vi "TxtToEye.vi"() -> ()   [LabVIEW 2022 SP3]
uses:
  <vilib>/Utility/file.llb/Read From Spreadsheet File (DBL).vi
  <vilib>/Analysis/NI_AALBase.lvlib
  <vilib>/Analysis/baseanly.llb/Quick Scale 2D.vi
panel:
  in  "Dig Word Size":u16
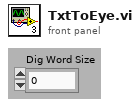
[diagram p1: front panel]
types:
  T1 = enum16{"big-endian, network order", "native, host order", "little-endian"}
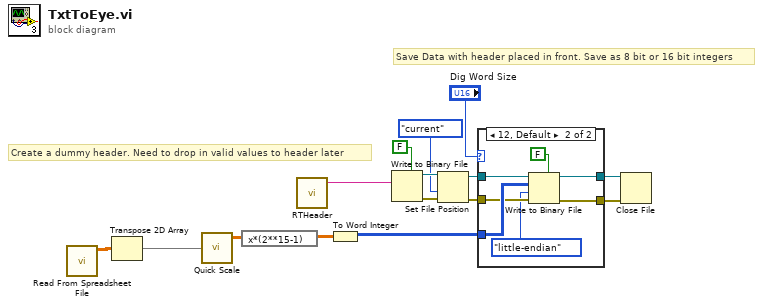
[diagram p0: block diagram]
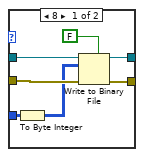
[diagram p2: hidden frame]
diagram:
  # "Create a dummy header. Need to drop in valid values to header later"
  # "Save Data with header placed in front. Save as 8 bit or 16 bit integers"
  n1 = call-poly <vilib>:"Read From Spreadsheet File.vi"() -> ("all rows"=w15:dbl[][])  [unwired: 7 in, 4 out]
  n2 = Transpose 2D Array(2D array=w15) -> (transposed array=w2:dbl[][])
  n3 = call-poly <vilib>:"Quick Scale.vi"("X"=w2) -> ("Yij=Xij/Max|X|"=w14:dbl[][])  [unwired: 2 out]
  n4 = expression code="x*(2**15-1)"(w14) -> (w13:dbl[][])
  n5 = call "RTHeader.vi"() -> ("Header String Out"=w1:string)  [unwired: 3 in, 2 out]
  n6 = To Word Integer(number=w13) -> (16bit integer=w3:i16[][])
  n7 = Write to Binary File(data=w1, 5:FALSE ("prepend array or string size? (T)")) -> (refnum out=w10:refnum<file>, error out=w9:errorcluster)  [unwired: 2 in, 3 out]
  n8 = Set File Position(refnum=w10, from (0:start)=enum16{"start", "end", "current"}."current" ("pos mode (0:2)"), error in=w9) -> (refnum out=w7:refnum<file>, error out=w6:errorcluster)  [unwired: 1 out]
  n9 = case shown="12, Default" "Dig Word Size" {
    tunnel: w3 -> [w18 w29]
    tunnel: w7 -> [w22 w28]
    tunnel: w6 -> [w21 w27]
    tunnel: [w20 w26] -> w5
    tunnel: [w19 w25] -> w4
    frame 8 {
      n10 = To Byte Integer(number=w18) -> (8bit integer=w16:i8[][])
      n11 = Write to Binary File(file (use dialog)=w22, data=w16, error in=w21, 5:FALSE) -> (refnum out=w20:refnum<file>, error out=w19:errorcluster)  [unwired: 1 in, 2 out]
    }
    frame 12, Default {
      n12 = Write to Binary File(file (use dialog)=w28, data=w29, error in=w27, 5:FALSE ("prepend array or string size? (T)"), 9:T1."little-endian" ("byte order (0:big-endian, network order)")) -> (refnum out=w26:refnum<file>, error out=w25:errorcluster)  [unwired: 2 out]
    }
  }
  n13 = Close File(refnum=w5, error in=w4) -> ()  [unwired: 2 out]
